vi "PromptForProjNum.vi"() -> (0 "ProjectNumber OUT":string caption="ProjectNumber")   [LabVIEW 2016]
doc: "Displays a standard dialog box that prompts users to enter information, such as a user name and password.\n--------------------\n\nThis Express VI is configured as follows:\n\nMessage to Display to the User:Project Number is required in order to file results correctly. Please enter the Project Number\nThe inputs are: \nText Entry Box: ProjectNumber"
uses:
  ADAM Client/Sub VIs/ADAM Controls/Ch_description_ADAM.ctl
  ADAM Client/Sub VIs/ADAM Controls/Module_type_ADAM.ctl
  ADAM Client/Sub VIs/ADAM Controls/Function_ADAM.ctl
  ADAM Client/Sub VIs/ADAM Controls/Channel_State.ctl
  ADAM Client/Sub VIs/ADAM Controls/Calib_type_ADAM.ctl
  ADAM Client/Sub VIs/ADAM Controls/Address.ctl
  ADAM Client/Sub VIs/ADAM Controls/Update_scan_value.ctl
  Globals/Preference_global.vi
panel:
  out "End":bool
  out "Startup":bool
  in  "ProjectNumber":string
  in  "OK":bool caption="OK1"
  # "Project Number is required in order to file results correctly.\nPlease enter the Project Number :"
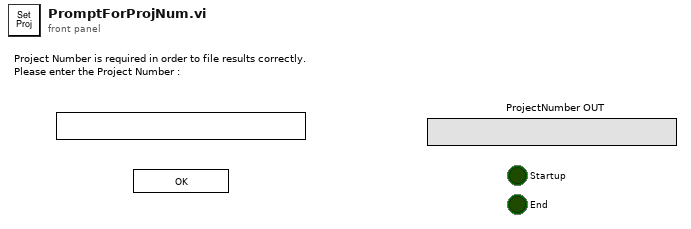
[diagram p1: front panel]
types:
  T1 = typedef "Ch_description_ADAM.ctl" = cluster{"Ch Name":string, "Type":T2, "Function":T3, "Ch State":T4, "Calibration type":T5, "A":dbl, "B":dbl, "C":dbl, "D":dbl, "Comments":string, "Address":T6, "String":string, "Duty":u16}
  T2 = typedef "Module_type_ADAM.ctl" = string
  T3 = typedef "Function_ADAM.ctl" = enum16{"Analogue Input", "Digital Input", "Event counter", "Event rate", "Analogue Output", "Digital Output", "Relay Output"}
  T4 = typedef "Channel_State.ctl" = enum16{"On", "Off", "Always On", "Always Off"}
  T5 = typedef "Calib_type_ADAM.ctl" = enum16{"Raw", "Bx + A", "Cx^2 + Bx + A", "Dx^3 + Cx^2 + Bx + A", "In Band", "Hi-Tec Q", "Hi-Tec M_dot", "Text"}
  T6 = typedef "Address.ctl" = cluster{"Main":i32, "Ch.":i32, "Sub":i32, "Port Name":string}
  T7 = typedef "Update_scan_value.ctl" = cluster{"Channel Name":string, "New Value":dbl}
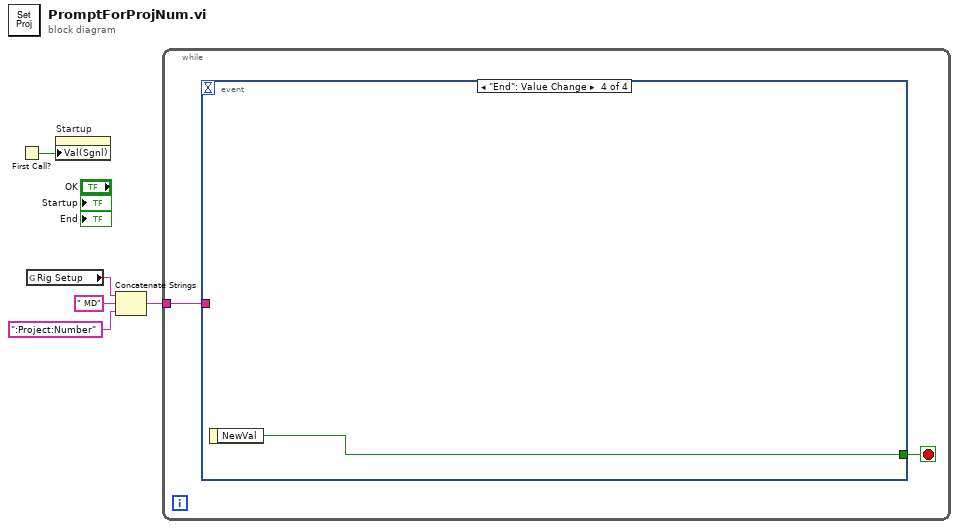
[diagram p0: block diagram]
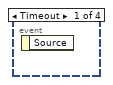
[diagram p2: hidden frame]
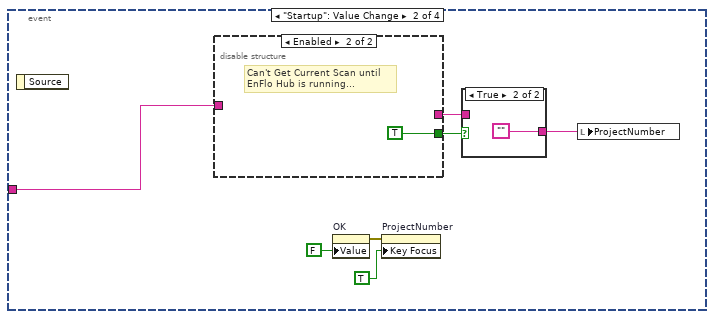
[diagram p3: hidden frame]
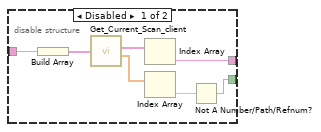
[diagram p4: hidden frame]
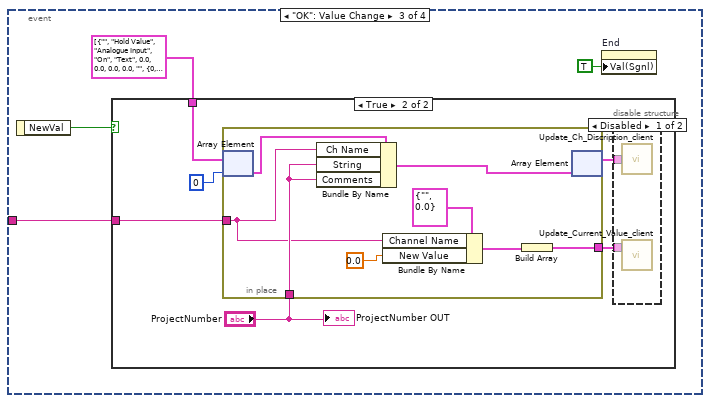
[diagram p6: hidden frame]
diagram:
  n1 = First Call?() -> (First Call?: T/F=w5:bool)
  n2 = global read "Preference_global.vi" "Rig Setup"() -> (w2:string)
  n3 = property on="Startup" class="Bool (strict)"("Val(Sgnl)"=w5) -> ()  [unwired: 2 in, 2 out]
  n4 = Concatenate Strings(w2, " MD", ":Project:Number") -> (w1:string)
  n5 = while {
    tunnel: w1 -> [w7]
    stop <- w6 stop-if-true
    n6 = event shown="[3] \"End\": Value Change" {
      selector: _ -> [_ _ _ _]
      dyn-events: _ -> [_ _ _ _]
      timeout: _ -> [_ _ _ _]
      tunnel: w7 -> [_ w14 w25 _]
      tunnel: [_ _ _ w45] -> w6
      event Timeout {
        n7 = event-data() -> ()  [unwired: 1 in, 1 out]
      }
      event "Startup": Value Change {
        n8 = event-data() -> ()  [unwired: 1 in, 1 out]
        n9 = disable-structure shown="Enabled" {
          disable-tunnel: w14 -> [w21 _]
          disable-tunnel: [w16 TRUE] -> w10
          disable-tunnel: [w15 _] -> w8
          frame Disabled {
            n10 = Build Array(w21) -> (w20:string[])
            n11 = call "Get_Current_Scan_client.vi"("ADAM Ch Names"=w20) -> ("String values"=w19:string[], "Numerical Values"=w18:dbl[])  [unwired: 2 out]
            n12 = Index Array(array=w19) -> (element=w15:string)  [unwired: 1 in]
            n13 = Index Array(array=w18) -> (element=w17:dbl)  [unwired: 1 in]
            n14 = Not A Number/Path/Refnum?(number/path/refnum=w17) -> (NaN/Path/Refnum?=w16:bool)
          }
          frame Enabled {
            # "Can't Get Current Scan until\nEnFlo Hub is running..."
          }
        }
        n15 = property on="OK" class="Bool (strict)"("Value"=FALSE ("OK")) -> (error out=w11:errorcluster)  [unwired: 2 in, 1 out]
        n16 = property on="ProjectNumber" class="Str"(error in=w11, "Key Focus"=TRUE ("focus on")) -> ()  [unwired: 1 in, 2 out]
        n17 = case shown="True" w10 {
          tunnel: [w23 ""] -> w9
          tunnel: w8 -> [w23 _]
          frame False {
          }
          frame True {
          }
        }
        n18 = local write "ProjectNumber"(w9) -> ()
      }
      event "OK": Value Change {
        n19 = event-data() -> ("NewVal"=w28:bool)  [unwired: 1 in]
        n20 = case shown="True" w28 {
          tunnel: T1[] [{"Ch Name"="", "Type"="Hold Value", "Function"=enum."Analogue Input", "Ch State"=enum."On", "Calibration type"=enum."Text", "A"=0.0, "B"=0.0, "C"=0.0, "D"=0.0, "Comments"="", "Address"={"Main"=0, "Ch."=0, "Sub"=0, "Port Name"=""}, "String"="", "Duty"=0}] ("Ch Description Array") -> [_ w34]
          tunnel: w25 -> [_ w29]
          frame False {
          }
          frame True {
            n21 = in-place {
              in-place-border: "ProjectNumber" -> [w44]
              in-place-border: [w39] -> w33
              in-place-border: w29 -> [w37]
              n22 = in-place-array #1(w34, 0) -> (w42:T1)
              n23 = Bundle By Name(cluster=w42, "Ch Name"=w37, "String"=w44, "Comments"=w44) -> (w41:T1)
              n24 = Bundle By Name(cluster=T7 {"Channel Name"="", "New Value"=0.0} ("Update Scan Value Cluster"), "Channel Name"=w37, "New Value"=0.0) -> (w40:T7)
              n25 = Build Array(w40) -> (w39:T7[])
              n26 = in-place-array #1(w41) -> (w32:T1[])  [unwired: 1 out]
            }
            n27 = disable-structure shown="Disabled" {
              disable-tunnel: w33 -> [w36 _]
              disable-tunnel: w32 -> [w35 _]
              frame Disabled {
                n28 = call "Update_Ch_Discription_client.vi"("Channels to update In"=w35) -> ()  [unwired: 1 out]
                n29 = call "Update_Current_Value_client.vi"("Update array in"=w36) -> ()  [unwired: 1 in]
              }
              frame Enabled {
              }
            }
            "ProjectNumber OUT" <- "ProjectNumber"
          }
        }
        n30 = property on="End" class="Bool (strict)"("Val(Sgnl)"=TRUE ("Value (Signaling)")) -> ()  [unwired: 2 in, 2 out]
      }
      event "End": Value Change {
        n31 = event-data() -> ("NewVal"=w45:bool)  [unwired: 1 in]
      }
    }
  }
